vi "FRAS Modes.vi"(0 "FRAS_Mode":T1(ring), 5 "CdG(t)":dbl[](array[numeric]), 7 "CdG res":dbl[](array[numeric]), 9 "Gain_int":dbl) -> (6 "CdG(t+1)":dbl[](array[numeric]), 10 "CdG commande":dbl[](array[numeric]))   [LabVIEW 2020]
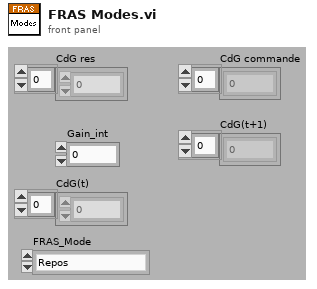
[diagram p1: front panel]
types:
  T1 = enum16{"Repos", "Détection", "Acquisition", "Poursuite", "Poursuite en a", "Poursuite en b"}
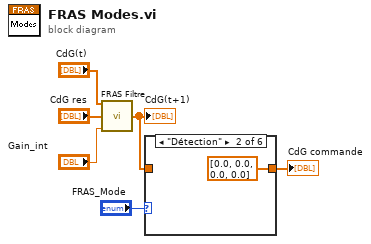
[diagram p0: block diagram]
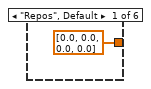
[diagram p2: hidden frame]
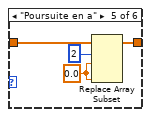
[diagram p5: hidden frame]
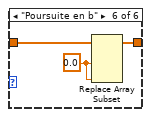
[diagram p6: hidden frame]
diagram:
  n1 = call "FRAS Filtre.vi"("CdG(t)"="CdG(t)", "Tableau 2"="CdG res", "Gain_int"="Gain_int") -> ("Tableau"=w4:dbl[])  [unwired: 12 out]
  "CdG(t+1)" <- w4
  n2 = case shown="\"Détection\"" "FRAS_Mode" {
    tunnel: w4 -> [_ _ w9 w10 w13 w17]
    tunnel: [dbl[] [0.0, 0.0, 0.0, 0.0] ("Tableau") dbl[] [0.0, 0.0, 0.0, 0.0] ("Tableau") w9 w10 w14 w16] -> w5
    frame "Repos", Default {
    }
    frame "Détection" {
    }
    frame "Acquisition" {
    }
    frame "Poursuite" {
    }
    frame "Poursuite en a" {
      w11 = 0.0
      n3 = Replace Array Subset(array=w13, new element #1=w11, index #1=2 ("indice"), new element #2=w11) -> (w14:dbl[])  [unwired: 1 in]
    }
    frame "Poursuite en b" {
      w15 = 0.0
      n4 = Replace Array Subset(array=w17, new element #1=w15, new element #2=w15) -> (w16:dbl[])  [unwired: 2 in]
    }
  }
  "CdG commande" <- w5
